vi "Lockin.Client.vi"(8 "error in (no error)":errorcluster, 9 "Data":variant, 10 "Command":T1, 11 "Instrument.Lockin in":refnum<class "Instrument.Lockin.lvclass">) -> (0 "error out":errorcluster, 1 "Data out":variant, 3 "Instrument.Lockin out":refnum<class "Instrument.Lockin.lvclass">)   [LabVIEW 2020, in "Instrument.Lockin.lvclass"]
uses:
  Instrument.Lockin.lvclass
  C:/Program Files (x86)/National Instruments/LabVIEW 2020/user.lib/LevyLab/Levylab Instruments/SMOs/Instrument/Instrument.lvclass
  Instrument.Lockinl.UI/Typedefs/Lockin.Commands--Enum.ctl
  <userlib>/LevyLab/Levylab Instruments/SMOs/Instrument/Instrument.lvclass
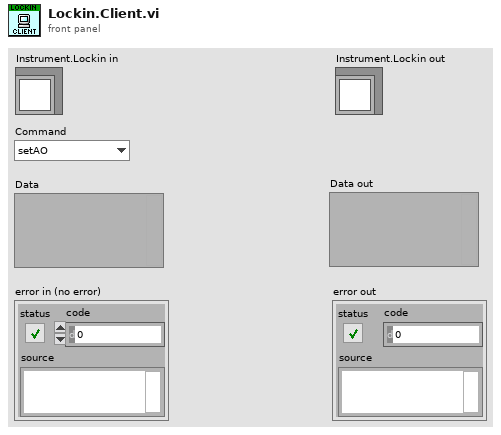
[diagram p1: front panel]
types:
  T1 = typedef "Instrument.Lockin.lvclass/Lockin.Commands--Enum.ctl" = enum16{"setAO", "setAO_Amplitude", "setAO_DC", "setAO_Frequency", "setAO_Phase", "setAO_Function", "setAO_I+", "setREF", "setREF_Frequency", "setREF_Phase", "setIVmode", "setAIDAQ", "setAODAQ", "Reset", "setSampling", "Trigger", "getAO", "getAI", "getResults", "getTrigger", "getIVmode", "getSampling", "getAOconfig", "getREFconfig", "setGain", "getGain", "setAutoSampling", "getAutoSampling", "setSweep", "getStatus", "getSweepResults", "getIVSweepResults", "startSweep", "stopSweep", "setAUX", "getAUX", "getRefreshTime"}
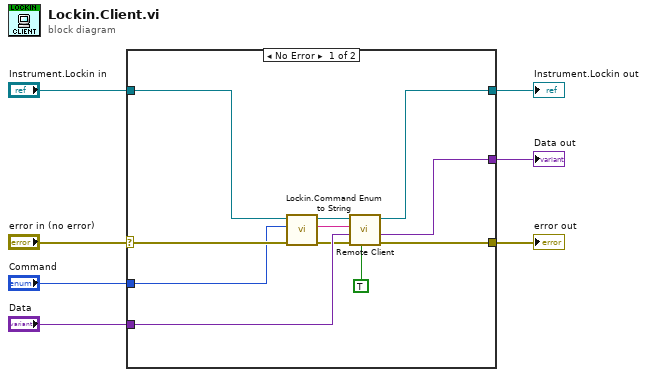
[diagram p0: block diagram]
diagram:
  n1 = case shown="No Error" "error in (no error)" {
    selector: "error in (no error)" -> [w12 w20]
    tunnel: "Data" -> [w18 _]
    tunnel: [w17 w20] -> w6
    tunnel: [w16 _] -> w5
    tunnel: "Command" -> [w9 _]
    tunnel: "Instrument.Lockin in" -> [w8 w19]
    tunnel: [w14 w19] -> w1
    frame No Error {
      n2 = call "Lockin.Command Enum to String.vi"("error in (no error)"=w12, "Command"=w9, "Instrument.Lockin in"=w8) -> ("error out"=w11:errorcluster, "Command"=w13:string, "Instrument.Lockin out"=w10:refnum<class "Instrument.Lockin.lvclass">)  [unwired: 5 in, 1 out]
      n3 = call <userlib>:"Remote Client.vi"("Wait for Response? [T]"=TRUE ("Wait for Response?"), "error in (no error)"=w11, "Data"=w18, "Command"=w13, "Instrument in"=w10) -> ("error out"=w17:errorcluster, "Data out"=w16:variant, "Instrument out"=w14:refnum<class "Instrument.Lockin.lvclass">)  [unwired: 3 in, 1 out]
    }
    frame Error {
    }
  }
  "Instrument.Lockin out" <- w1
  "error out" <- w6
  "Data out" <- w5
